vi "COMI US File Convert.vi"(9 "nMaxDataRow":u32, 10 "szTextFilePath":string, 11 "szBinFilePath":string) -> (2 "szTextFilePath out":string, 3 "szBinFilePath out":string)   [LabVIEW 2017, in "Comidll.lvlib"]
doc: "void (COMI_US_FileConvert) (char *szBinFilePath, char *szTextFilePath, unsigned long nMaxDataRow);"
uses:
  <userlib>/Comidll/Comidll.lvlib
  <userlib>/Comidll/Comidll.dll
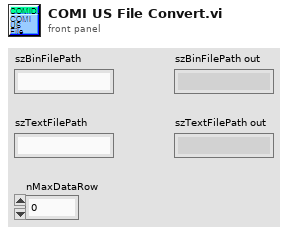
[diagram p1: front panel]
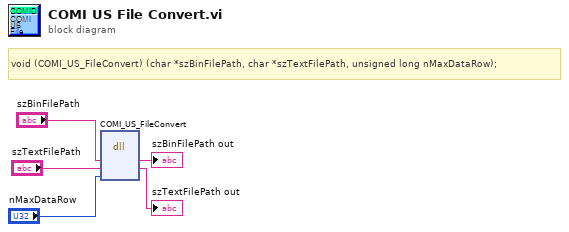
[diagram p0: block diagram]
diagram:
  # "void\t(COMI_US_FileConvert) (char *szBinFilePath, char *szTextFilePath, unsigned long nMaxDataRow);"
  n1 = dll-call lib="C:/Program Files/National Instruments/LabVIEW 2017/user.lib/Comidll/Comidll.*" fn="COMI_US_FileConvert"("szBinFilePath"="szBinFilePath", "szTextFilePath"="szTextFilePath", "nMaxDataRow"="nMaxDataRow") -> ("szBinFilePath"=→"szBinFilePath out":string, "szTextFilePath"=→"szTextFilePath out":string)  [unwired: 5 in, 2 out]
